vi "Curseur Create.vi"(8 "error in (no error)":errorcluster caption="entrée d'erreur (pas d'erreur)", 9 "Data Cam Processing":T1 {"sigma X" format="%0.2f"; "mean X" format="%0.2f"; "mean Y" format="%0.2f"; "sigma Y" format="%0.2f"; "Shutter (us)" scale=22.0..10000000.0; "Gain Caméra" scale=0.0..1023.0}, 10 "Curseur":T3) -> (0 "error out":errorcluster caption="sortie d'erreur", 1 "Data Cam Processing out":T1 {"sigma X" format="%0.2f"; "mean X" format="%0.2f"; "mean Y" format="%0.2f"; "sigma Y" format="%0.2f"; "Shutter (us)" scale=22.0..10000000.0; "Gain Caméra" scale=0.0..1023.0}, 2 "Img ROI":i16[][](array[numeric]), 3 "Image Out":i16[][](array[numeric]))   [LabVIEW 2026]
uses:
  Data-Processing.ctl
  <vilib>/Serenial/G Industrial Camera/g_industrial_cam/Buffer/Buffer.lvclass
  <vilib>/Serenial/G Industrial Camera/g_industrial_cam/Camera/Camera.lvclass
  <vilib>/picture/picture.llb/imagedata.ctl
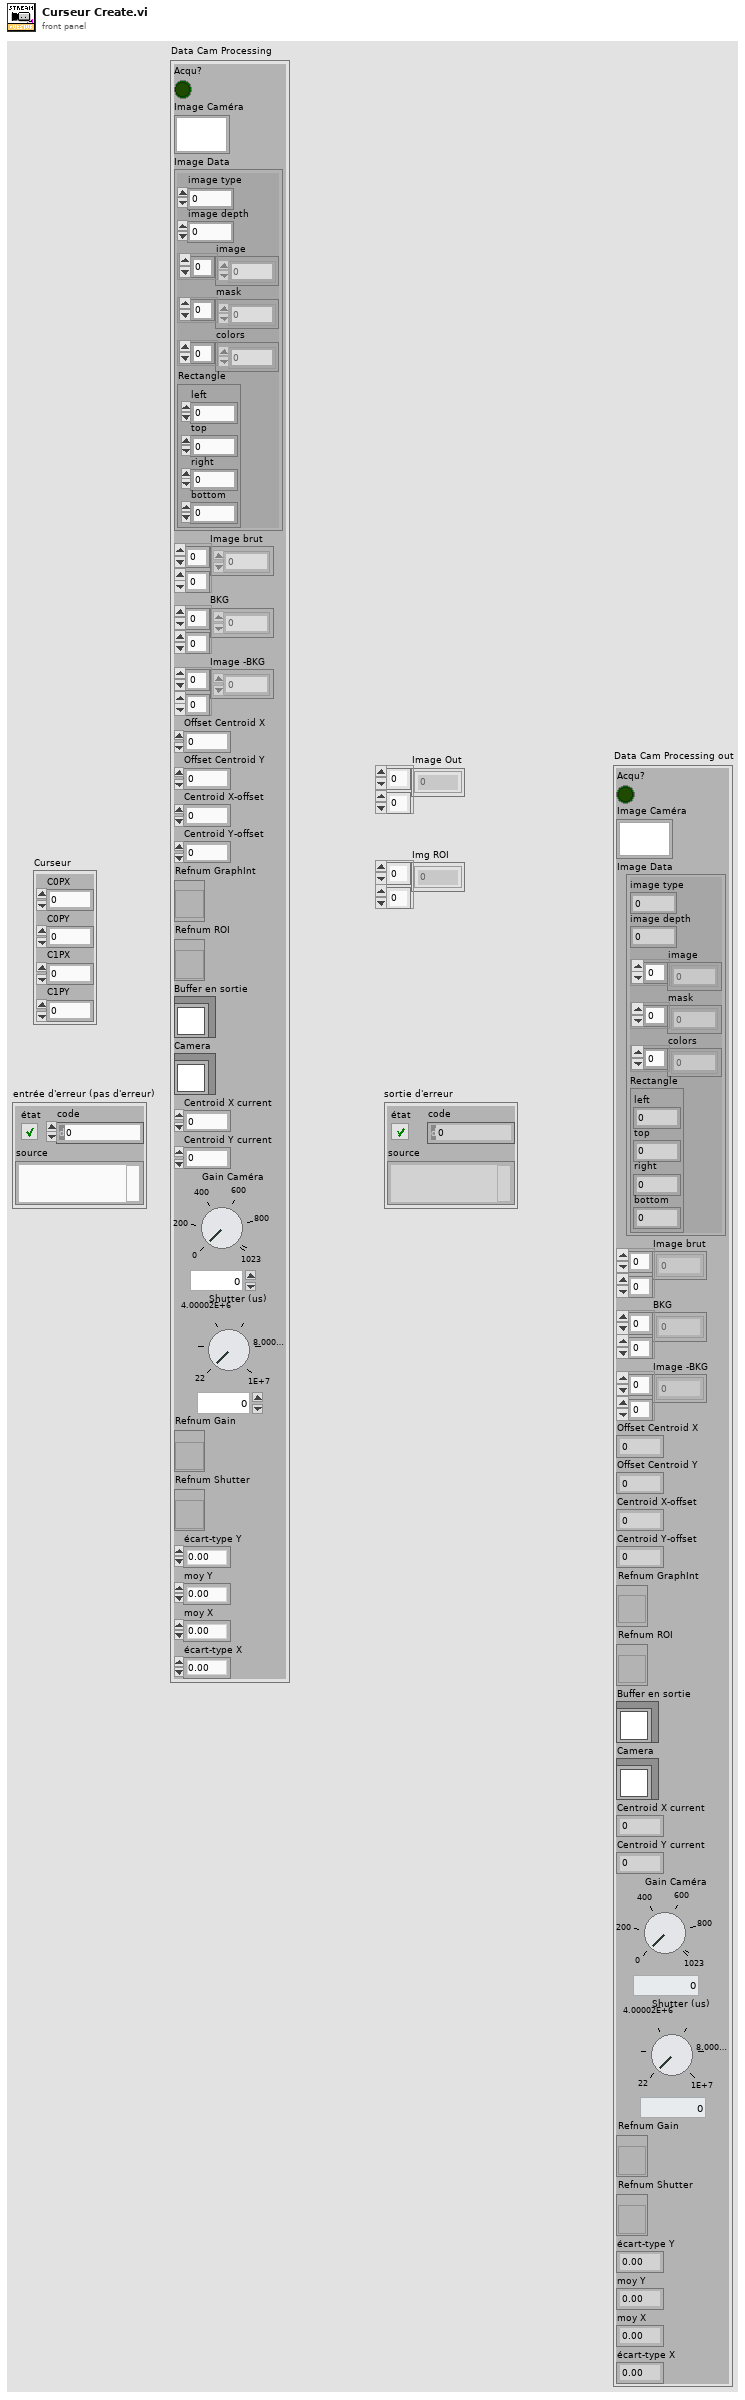
[diagram p1: front panel]
types:
  T1 = typedef "Data-Processing.ctl" = cluster{"Acqu?":bool, "Image Caméra":picture, "Image Data":T2, "Image brut":i16[][], "BKG":i16[][], "Image -BKG":i16[][], "Offset Centroid X":dbl, "Offset Centroid Y":dbl, "Centroid X-offset":dbl, "Centroid Y-offset":dbl, "Refnum GraphInt":refnum<vi>, "Refnum ROI":refnum<vi>, "Buffer en sortie":refnum<class "Buffer.lvclass">, "Camera":refnum<class "Camera.lvclass">, "Centroid X current":dbl, "Centroid Y current":dbl, "Gain Caméra":i32, "Shutter (us)":dbl, "Refnum Gain":refnum<vi>, "Refnum Shutter":refnum<vi>, "sigma Y":dbl, "mean Y":dbl, "mean X":dbl, "sigma X":dbl}
  T2 = typedef "imagedata.ctl" = cluster{"image type":i32, "image depth":i32, "image":u8[], "mask":u8[], "colors":u32[], "Rectangle":cluster{"left":i16, "top":i16, "right":i16, "bottom":i16}}
  T3 = cluster{"C0PX":dbl, "C0PY":dbl, "C1PX":dbl, "C1PY":dbl}
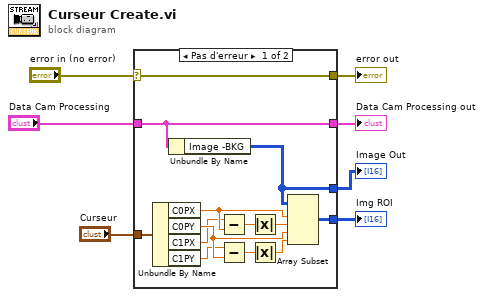
[diagram p0: block diagram]
diagram:
  n1 = case shown="Pas d'erreur" "error in (no error)" {
    selector: "error in (no error)" -> [w10 w22]
    tunnel: [w20 _] -> w7
    tunnel: "Curseur" -> [w11 _]
    tunnel: [w10 w22] -> w4
    tunnel: [w8 _] -> w3
    tunnel: [w9 w21] -> w2
    tunnel: "Data Cam Processing" -> [w9 w21]
    frame No Error {
      n2 = Unbundle By Name(w11) -> ("C0PX"=w13:dbl, "C0PY"=w17:dbl, "C1PX"=w12:dbl, "C1PY"=w16:dbl)
      n3 = Unbundle By Name(w9) -> ("Image -BKG"=w8:i16[][])
      n4 = Subtract(x=w12, y=w13) -> (x-y=w14:dbl)
      n5 = Subtract(x=w16, y=w17) -> (x-y=w18:dbl)
      n6 = Absolute Value(x=w14) -> (abs(x)=w15:dbl)
      n7 = Absolute Value(x=w18) -> (abs(x)=w19:dbl)
      n8 = Array Subset(array=w8, index (row)=w13, length (row)=w15, index (col)=w17, length (col)=w19) -> (w20:i16[][])
    }
    frame Error {
    }
  }
  "Img ROI" <- w7
  "Image Out" <- w3
  "error out" <- w4
  "Data Cam Processing out" <- w2
